vi "add_3d_arrays.vi"(6 "error in":errorcluster, 8 "3d array in 2":dbl[][][](array[numeric]), 9 "3d arry in 1":dbl[][][](array[numeric])) -> (0 "error out":errorcluster, 3 "3d array sum out":dbl[][][](array[numeric]))   [LabVIEW 2011, in "Fiberscope_library.lvlib"]
uses:
  Fiberscope_library.lvlib
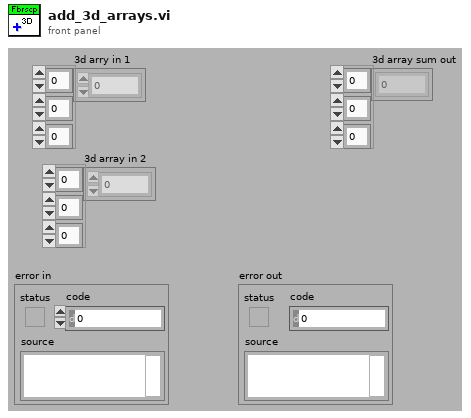
[diagram p1: front panel]
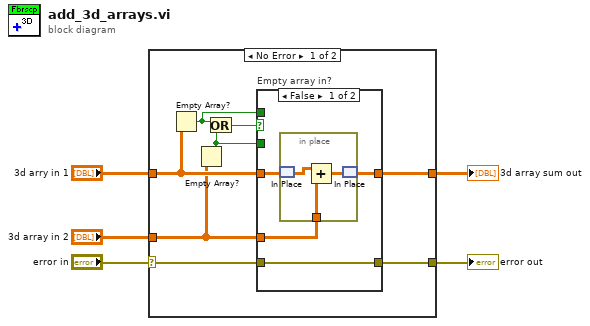
[diagram p0: block diagram]
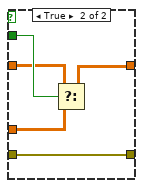
[diagram p2: hidden frame]
diagram:
  n1 = case shown="No Error" "error in" {
    selector: "error in" -> [w10 w27]
    tunnel: [w9 w27] -> w4
    tunnel: [w13 w26] -> w2
    tunnel: "3d arry in 1" -> [w12 w26]
    tunnel: "3d array in 2" -> [w11 _]
    frame No Error {
      n2 = Empty Array?(array=w12) -> (empty?=w7:bool)
      n3 = Empty Array?(array=w11) -> (empty?=w6:bool)
      n4 = Or(x=w7, y=w6) -> (x .or. y?=w8:bool)
      n5 = case "Empty array in?" shown="False" w8 {
        tunnel: w11 -> [w16 w24]
        tunnel: w12 -> [w15 w23]
        tunnel: [w14 w22] -> w13
        tunnel: [w17 w21] -> w9
        tunnel: w10 -> [w17 w21]
        tunnel: w7 -> [_ _]
        tunnel: w6 -> [_ w25]
        frame False {
          n6 = in-place {
            in-place-border: w16 -> [w20]
            n7 = in-place-match #1(w15) -> (w19:dbl[][][])
            n8 = Add(x=w19, y=w20) -> (x+y=w18:dbl[][][])
            n9 = in-place-match #1(w18) -> (w14:dbl[][][])
          }
        }
        frame True {
          n10 = Select(t=w23, s=w25, f=w24) -> (s? t:f=w22:dbl[][][])
        }
      }
    }
    frame Error {
    }
  }
  "3d array sum out" <- w2
  "error out" <- w4
